vi "Read Output.vi"(8 "error in":errorcluster, 11 "GEN40-38-LAN in":refnum<class "GEN40-38-LAN.lvclass">) -> (0 "error out":errorcluster, 2 "Output":bool, 3 "GEN40-38-LAN out":refnum<class "GEN40-38-LAN.lvclass">)   [LabVIEW 2018, in "GEN40-38-LAN.lvlib" / "GEN40-38-LAN.lvclass"]
uses:
  GEN40-38-LAN.lvclass
  PPLs/Power Supply/Parent/Power_Supply.lvlibp/Power Supply.lvclass
  C:/Projects/LabVIEW/PPLs/Power Supply/Parent/Power_Supply.lvlibp/Power Supply.lvclass
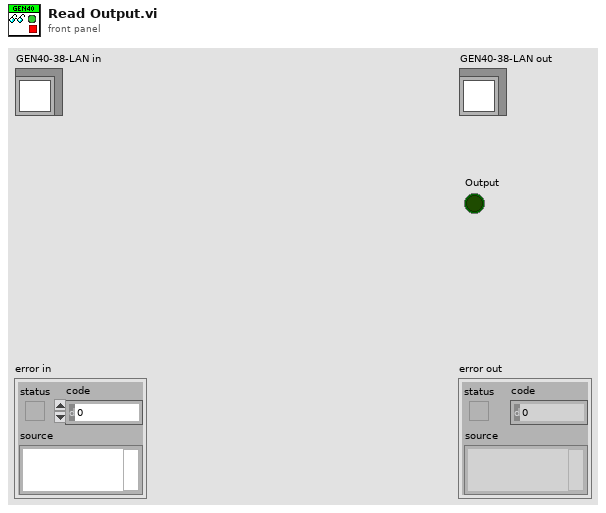
[diagram p1: front panel]
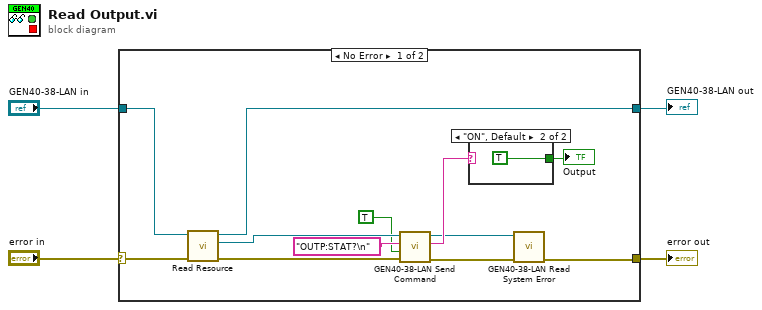
[diagram p0: block diagram]
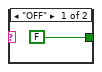
[diagram p2: hidden frame]
diagram:
  n1 = case shown="No Error" "error in" {
    selector: "error in" -> [w5 w20]
    tunnel: [w6 w20] -> w3
    tunnel: [w14 w19] -> w4
    tunnel: "GEN40-38-LAN in" -> [w16 w19]
    frame No Error {
      n2 = call "Read Resource.vi"("error in"=w5, "Power Supply in"=w16) -> ("error out"=w15:errorcluster, "Resource"=w13:refnum<visa-resource-name>, "Power Supply out"=w14:refnum<class "GEN40-38-LAN.lvclass">)  [unwired: 7 in]
      n3 = call "GEN40-38-LAN Send Command.vi"("error in (no error)"=w15, "Wait for Response?"=TRUE, "Command"="OUTP:STAT?\n", "VISA resource name"=w13) -> ("error out"=w7:errorcluster, "Response"=w9:string, "VISA resource name out"=w8:refnum<visa-resource-name>)  [unwired: 5 in]
      n4 = case shown="\"ON\", Default" w9 {
        tunnel: [FALSE TRUE] -> w10
        frame "OFF" {
        }
        frame "ON", Default {
        }
      }
      "Output" <- w10
      n5 = call "GEN40-38-LAN Read System Error.vi"("error in (no error)"=w7, "Resource"=w8) -> ("error out"=w6:errorcluster)  [unwired: 9 in]
    }
    frame Error {
    }
  }
  "error out" <- w3
  "GEN40-38-LAN out" <- w4
